vi "Dual Joystick Drive.vi"(0 "Joystick 1":T2, 1 "Joystick 2":T2) -> (2 "Strafe":dbl, 3 "Forward/Backward":dbl, 4 "Turn":dbl)   [LabVIEW 2013]
uses:
  <vilib>/Rock Robotics/WPI/Joystick/WPI_JoystickButtonState.ctl
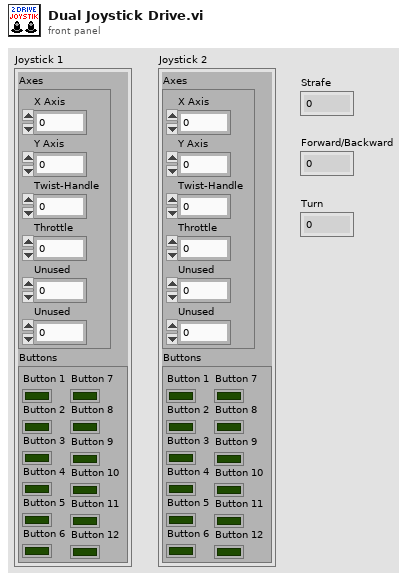
[diagram p1: front panel]
types:
  T1 = typedef "WPI_JoystickButtonState.ctl" = cluster{"Button 1":bool, "Button 2":bool, "Button 3":bool, "Button 4":bool, "Button 5":bool, "Button 6":bool, "Button 7":bool, "Button 8":bool, "Button 9":bool, "Button 10":bool, "Button 11":bool, "Button 12":bool}
  T2 = cluster{"Axes":cluster{"X Axis":dbl, "Y Axis":dbl, "Twist-Handle":dbl, "Throttle":dbl, "Unused":dbl, "Unused":dbl}, "Buttons":T1}
  T3 = cluster{"X Axis":dbl, "Y Axis":dbl, "Twist-Handle":dbl, "Throttle":dbl, "Unused":dbl, "Unused":dbl}
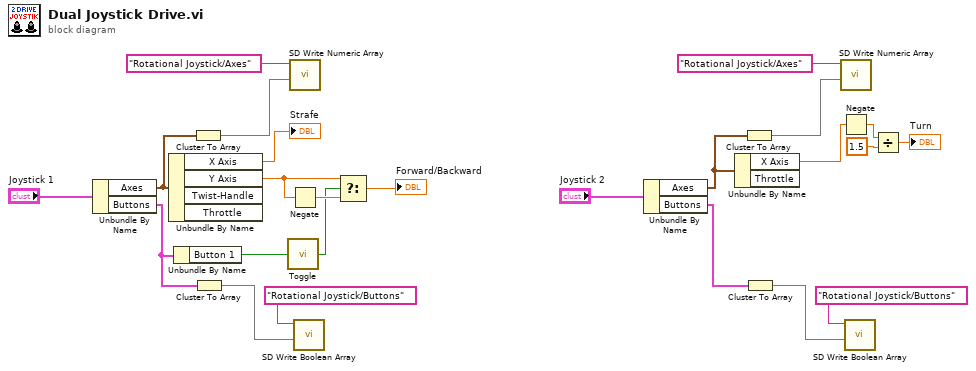
[diagram p0: block diagram]
diagram:
  n1 = Unbundle By Name("Joystick 1") -> ("Axes"=w21:T3, "Buttons"=w17:T1)
  n2 = Unbundle By Name(w21) -> ("X Axis"=→"Strafe":dbl, "Y Axis"=w15:dbl)  [unwired: 2 out]
  n3 = Unbundle By Name(w17) -> ("Button 1"=w14:bool)
  n4 = Cluster To Array(cluster=w21) -> (array=w22:dbl[])
  n5 = Cluster To Array(cluster=w17) -> (array=w18:bool[])
  n6 = call "Toggle.vi"("Input"=w14) -> ("Latched"=w13:bool)
  n7 = call <vilib>:"SD Write Numeric Array.vi"("Numeric Array"=w22, "Name"="Rotational Joystick/Axes") -> ()  [unwired: 8 in, 2 out]
  n8 = Negate(x=w15) -> (-x=w16:dbl)
  n9 = call <vilib>:"SD Write Boolean Array.vi"("Boolean Array"=w18, "Name"="Rotational Joystick/Buttons") -> ()  [unwired: 8 in, 2 out]
  n10 = Select(t=w15, s=w13, f=w16) -> (s? t:f=→"Forward/Backward":dbl)
  n11 = Unbundle By Name("Joystick 2") -> ("Axes"=w8:T3, "Buttons"=w3:T1)
  n12 = Unbundle By Name(w8) -> ("X Axis"=w1:dbl)  [unwired: 1 out]
  n13 = Cluster To Array(cluster=w8) -> (array=w9:dbl[])
  n14 = Cluster To Array(cluster=w3) -> (array=w4:bool[])
  n15 = call <vilib>:"SD Write Numeric Array.vi"("Numeric Array"=w9, "Name"="Rotational Joystick/Axes") -> ()  [unwired: 8 in, 2 out]
  n16 = Negate(x=w1) -> (-x=w6:dbl)
  n17 = call <vilib>:"SD Write Boolean Array.vi"("Boolean Array"=w4, "Name"="Rotational Joystick/Buttons") -> ()  [unwired: 8 in, 2 out]
  n18 = Divide(x=w6, y=1.5) -> (x/y=→"Turn":dbl)
